vi "imageQ_obtain.vi"() -> (0 "queue out":refnum<queue>)   [LabVIEW 2010]
uses:
  <vilib>/vision/Image Controls.llb/IMAQ Image.ctl
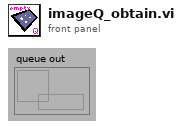
[diagram p1: front panel]
types:
  T1 = typedef "IMAQ Image.ctl" = refnum<image>
  T2 = cluster{"New Image":T1, "queue out":refnum<queue>}
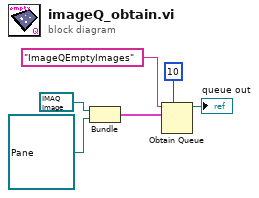
[diagram p0: block diagram]
diagram:
  n1 = Bundle("New Image"=T1 refnum, "queue out"=refnum<queue> refnum) -> (w2:T2)  [unwired: 1 in]
  n2 = Obtain Queue(max queue size (-1, unlimited)=10, name (unnamed)="ImageQEmptyImages", element data type=w2) -> (queue out=→"queue out":refnum<queue>)  [unwired: 2 in, 2 out]
